vi "Cleanup lib MPSSE.vi"(11 "error in (no error)":errorcluster) -> (15 "error out":errorcluster)   [LabVIEW 2017, in "libMPSSE.lvlib"]
doc: "FTDI_API void Cleanup_libMPSSE(void);"
uses:
  libMPSSE.lvlib
  \\Mac\Home/Desktop/libMPSSE-SPI-LabVIEW-master/libMPSSE.dll
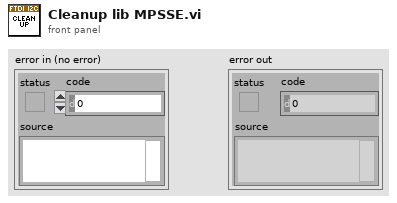
[diagram p1: front panel]
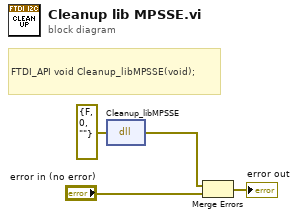
[diagram p0: block diagram]
diagram:
  # "FTDI_API void Cleanup_libMPSSE(void);"
  n1 = dll-call lib="\\\\Mac\\Home/Desktop/libMPSSE-SPI-LabVIEW-master/libMPSSE.dll" fn="Cleanup_libMPSSE"(error in=errorcluster {"status"=FALSE, "code"=0, "source"=""} ("error in (no error)")) -> (error out=w1:errorcluster)  [unwired: 3 in, 1 out]
  n2 = Merge Errors(w1, "error in (no error)") -> (→"error out":errorcluster)
